vi "LEP_RV_LoadProjectInfo.vi"(0 "TopLevelVIPath In":path, 11 "error in (no error)":errorcluster) -> (2 "Project File":path, 3 "Executable File":path, 4 "Status":T1(ring)=enum."EmptyTopLevelVIPath", 6 "TopLevelVIPath Out":path, 8 "Build Path":path, 10 "Target Name":string, 15 "error out":errorcluster)   [LabVIEW 2011]
doc: "Returns the build path of the LabVIEW Embedded Project in <B>TopLevelVIPath In</B>."
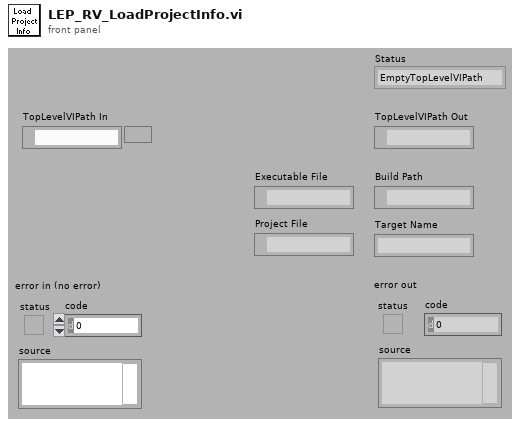
[diagram p1: front panel]
types:
  T1 = enum16{"NoErr", "TopLevelVIErr", "EmptyTopLevelVIPath", "CGenErr", "CpySuppFilesErr", "ProjectInfoErr", "NoTopLevelVIErr", "CreateBuildFolderErr", "EmptyBuildFolderErr", "LoadConfigErr", "BildToolsErr", "CompileErr", "LinkError", "DebugInfoErr", "NotFoundErr", "AccessErr", "ExecErr", "UnknownErr"}
  T2 = cluster{"KEIL Path":path, "Port Range Start":u16, "Port Range End":u16, "UV IP Address":string}
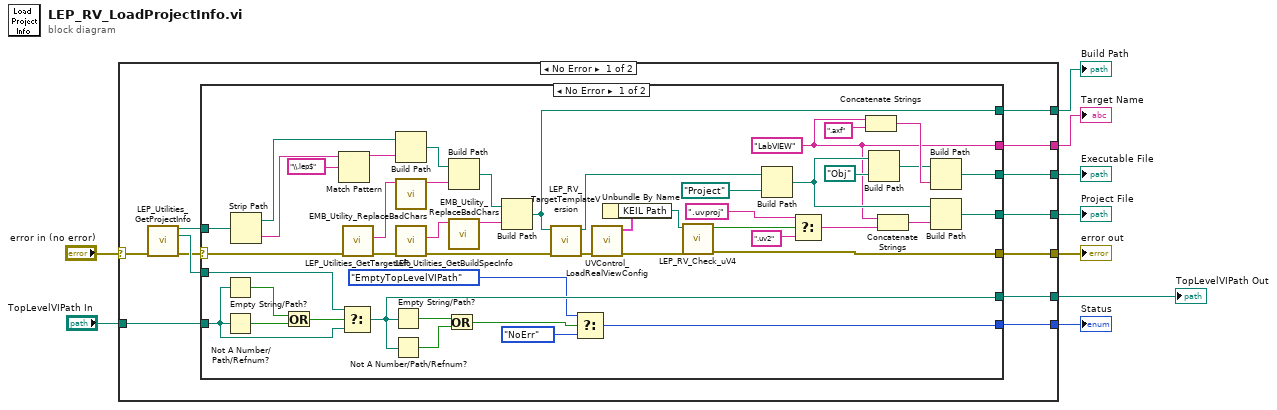
[diagram p0: block diagram]
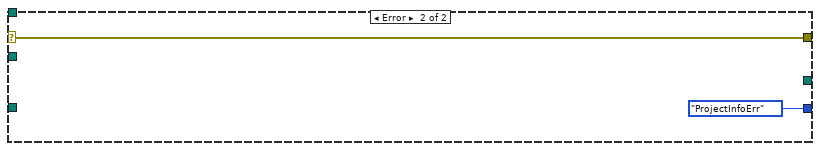
[diagram p2: hidden frame]
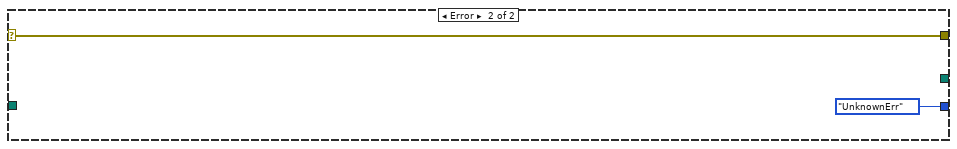
[diagram p3: hidden frame]
diagram:
  n1 = case shown="No Error" "error in (no error)" {
    selector: "error in (no error)" -> [w19 w72]
    tunnel: [w20 w72] -> w8
    tunnel: [w18 T1."UnknownErr" ("Errors")] -> w1
    tunnel: "TopLevelVIPath In" -> [w17 _]
    tunnel: [w16 _] -> w6
    tunnel: [w15 _] -> w5
    tunnel: [w14 _] -> w4
    tunnel: [w13 _] -> w3
    tunnel: [w12 _] -> w2
    frame No Error {
      n2 = call <vilib>:"LEP_Utilities_GetProjectInfo.vi"("error in"=w19) -> ("ProjectPath"=w10:path, "TopLevelVI"=w21:path, "error out"=w11:errorcluster)  [unwired: 10 in, 2 out]
      n3 = case shown="No Error" w11 {
        selector: w11 -> [w37 w70]
        tunnel: w21 -> [w65 _]
        tunnel: [w27 w70] -> w20
        tunnel: [w62 T1."ProjectInfoErr" ("Errors")] -> w18
        tunnel: w10 -> [w58 _]
        tunnel: w17 -> [w60 _]
        tunnel: [w59 _] -> w16
        tunnel: [w39 _] -> w15
        tunnel: [w33 _] -> w14
        tunnel: [w49 _] -> w13
        tunnel: [w43 _] -> w12
        frame No Error {
          w33 = "LabVIEW"
          n4 = Empty String/Path?(string/path=w60) -> (empty?=w67:bool)
          n5 = Not A Number/Path/Refnum?(number/path/refnum=w60) -> (NaN/Path/Refnum?=w68:bool)
          n6 = Strip Path(path=w58) -> (stripped path=w55:path, name=w57:string)
          n7 = Or(x=w67, y=w68) -> (x .or. y?=w66:bool)
          n8 = Match Pattern(string=w57, regular expression="\\.lep$") -> (before substring=w54:string)  [unwired: 1 in, 3 out]
          n9 = Select(t=w65, s=w66, f=w60) -> (s? t:f=w59:path)
          n10 = call <vilib>:"LEP_Utilities_GetTargetInfo.vi"("error in"=w37) -> ("error out"=w36:errorcluster, "display name"=w35:string)  [unwired: 7 in, 2 out]
          n11 = Empty String/Path?(string/path=w59) -> (empty?=w63:bool)
          n12 = Not A Number/Path/Refnum?(number/path/refnum=w59) -> (NaN/Path/Refnum?=w64:bool)
          n13 = Build Path(base path=w55, name or relative path=w54) -> (appended path=w53:path)
          n14 = call <vilib>:"EMB_Utility_ReplaceBadChars.vi"("Input String"=w35) -> ("Output String"=w34:string)  [unwired: 10 in]
          n15 = call <vilib>:"LEP_Utilities_GetBuildSpecInfo.vi"("error in"=w36) -> ("error out"=w40:errorcluster, "display name"=w32:string)  [unwired: 8 in, 1 out]
          n16 = Or(x=w63, y=w64) -> (x .or. y?=w61:bool)
          n17 = Build Path(base path=w53, name or relative path=w34) -> (appended path=w52:path)
          n18 = call <vilib>:"EMB_Utility_ReplaceBadChars.vi"("Input String"=w32) -> ("Output String"=w31:string)  [unwired: 10 in]
          n19 = Build Path(base path=w52, name or relative path=w31) -> (appended path=w39:path)
          n20 = call "LEP_RV_TargetTemplateVersion.vi"("error in (no error)"=w40, "Path"=w39) -> ("error out"=w25:errorcluster, "Path plus Version"=w38:path)  [unwired: 7 in, 1 out]
          n21 = Select(t=T1."EmptyTopLevelVIPath" ("Errors"), s=w61, f=T1."NoErr" ("Errors")) -> (s? t:f=w62:T1)
          n22 = call "UVControl_LoadRealViewConfig.vi"("error in (no error)"=w25) -> ("uVisionConfig"=w23:T2, "error out"=w24:errorcluster)  [unwired: 11 in, 2 out]
          n23 = Unbundle By Name(w23) -> ("KEIL Path"=w22:path)
          n24 = call "LEP_RV_Check_uV4.vi"("error in (no error)"=w24, "KEIL Path"=w22) -> ("error out"=w27:errorcluster, "uv4 installed"=w30:bool)  [unwired: 8 in]
          n25 = Build Path(base path=w38, name or relative path=path "Project") -> (appended path=w48:path)
          n26 = Select(t=".uvproj" ("string"), s=w30, f=".uv2") -> (s? t:f=w28:string)
          n27 = Concatenate Strings(w33, ".axf" ("string")) -> (w45:string)
          n28 = Build Path(base path=w48, name or relative path=path "Obj") -> (appended path=w44:path)
          n29 = Concatenate Strings(w33, w28) -> (w50:string)
          n30 = Build Path(base path=w44, name or relative path=w45) -> (appended path=w43:path)
          n31 = Build Path(base path=w48, name or relative path=w50) -> (appended path=w49:path)
        }
        frame Error {
        }
      }
    }
    frame Error {
    }
  }
  "error out" <- w8
  "TopLevelVIPath Out" <- w6
  "Build Path" <- w5
  "Target Name" <- w4
  "Executable File" <- w2
  "Project File" <- w3
  "Status" <- w1
